vi "Periodic Tasks.vi"(8 "error in":errorcluster) -> ()   [LabVIEW 2015]
doc: "This VI runs in parallel to other tasks. It can contain as many user-defined periodic loops as you need. These can carry out PID or other sorts of timed response."
uses:
  <vilib>/Rock Robotics/WPI/Utilities/WPI_GetSetVariantRefNum.vi
  <vilib>/Rock Robotics/SystemInterfaces/Utilities/FPGA_UtilitiesRead LocalTime.vi
  <vilib>/Rock Robotics/Network Tables/NT Write Number.vi
  <vilib>/Rock Robotics/Network Tables/NT Write Numeric Array.vi
panel:
  out "All PDP Currents":dbl[](array[numeric])
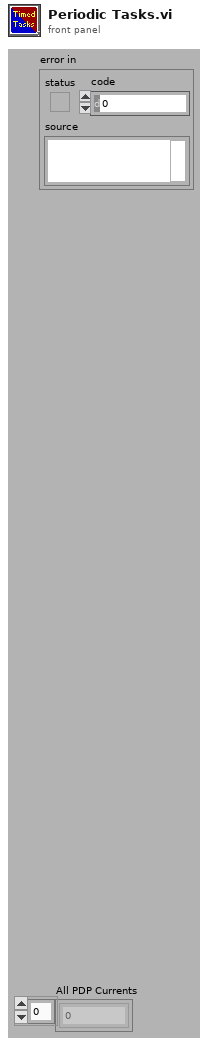
[diagram p1: front panel]
types:
  T1 = typedef "WPI_EncoderDevRef.ctl" = cluster{"DevStatus":errorcluster, "EncoderIndex":T2, "CounterIndex":T3, "DistancePerCount":dbl, "Decoding Type":T4}
  T2 = typedef "FPGA_EncoderIdx.ctl" = enum8{"Enc 0", "Enc 1", "Enc 2", "Enc 3", "Enc 4", "Enc 5", "Enc 6", "Enc 7", "Invalid"}
  T3 = typedef "FPGA_CounterCtrSystemIndex.ctl" = enum8{"Ctr 0", "Ctr 1", "Ctr 2", "Ctr 3", "Ctr 4", "Ctr 5", "Ctr 6", "Ctr 7", "Invalid"}
  T4 = typedef "WPI_EncoderType.ctl" = enum16{"1x", "2x", "4x"}
  T5 = typedef "WPI_JoystickDevRef.ctl" = cluster{"Device":T6}
  T6 = typedef "WPI_JoystickDeviceEnum.ctl" = enum16{"USB 0", "USB 1", "USB 2", "USB 3", "USB 4", "USB 5"}
  T7 = typedef "WPI_GyroDevRef.ctl" = cluster{"DevStatus":errorcluster, "Analog Channel":T8, "Offset":dbl, "Gain (VoltsPerDegree/Second)":dbl, "Gyro Type":enum16{"Analog", "XRS450"}, "Handle":i32, "SPI Bus":T9, "Device Found":bool, "Sample Rate":dbl, "Calibrate On Open":bool}
  T8 = typedef "FPGA_AIChannel.ctl" = enum8{"AI 0", "AI 1", "AI 2", "AI 3", "AI MXP 0", "AI MXP 1", "AI MXP 2", "AI MXP 3", "Invalid"}
  T9 = typedef "spi_bus.ctl" = enum16{"SPI On-Board, CS0", "SPI On-Board, CS1", "SPI On-Board, CS2", "SPI On-Board, CS3", "SPI MXP", "Invalid"}
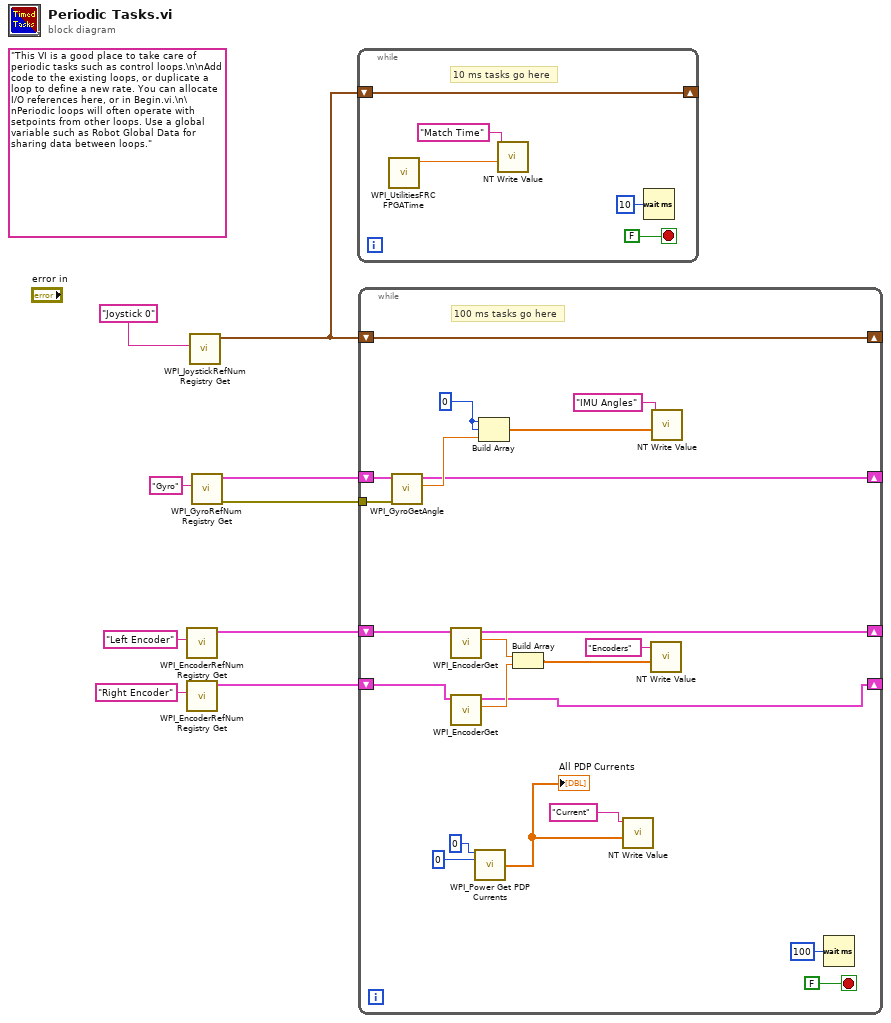
[diagram p0: block diagram]
diagram:
  (unwired) "This VI is a good place to take care of periodic tasks such as control loops.\n\nAdd code to the existing loops, or duplicate a loop to define a new rate. You can allocate I/O references here, or in Begin.vi.\n\nPeriodic loops will often operate with setpoints from other loops. Use a global variable such as Robot Global Data for sharing data between loops."
  n1 = call <vilib>:"WPI_EncoderRefNum Registry Get.vi"("refnum name"="Left Encoder") -> ("EncoderDevRef"=w5:T1)  [unwired: 9 in, 1 out]
  n2 = call <vilib>:"WPI_EncoderRefNum Registry Get.vi"("refnum name"="Right Encoder") -> ("EncoderDevRef"=w4:T1)  [unwired: 9 in, 1 out]
  n3 = call <vilib>:"WPI_JoystickRefNum Registry Get.vi"("refnum name"="Joystick 0") -> ("JoystickDevRef"=w8:T5)  [unwired: 1 in, 9 out]
  n4 = call <vilib>:"WPI_GyroRefNum Registry Get.vi"("refnum name"="Gyro") -> ("error out"=w3:errorcluster, "GyroDevRef"=w2:T7)  [unwired: 9 in]
  n5 = while {
    shift-right: [w12] -> _
    shift-left: w8 -> [w12]
    stop <- FALSE stop-if-true
    # "10 ms tasks go here"
    n6 = call <vilib>:"WPI_UtilitiesFRC FPGATime.vi"() -> ("FPGA Time"=w10:dbl)  [unwired: 10 in, 1 out]
    n7 = call-poly <vilib>:"NT Write Value.vi"("Numeric"=w10, "Name"="Match Time") -> ()  [unwired: 9 in, 1 out]
    n8 = Wait (ms)(milliseconds to wait=u32 10) -> ()  [unwired: 1 out]
  }
  n9 = while {
    shift-right: [w34] -> _
    shift-left: w8 -> [w34]
    shift-right: [w26] -> _
    shift-left: w5 -> [w28]
    shift-right: [w25] -> _
    shift-left: w4 -> [w27]
    tunnel: w3 -> [w19]
    shift-right: [w16] -> _
    shift-left: w2 -> [w15]
    stop <- FALSE stop-if-true
    w18 = 0
    # "100 ms tasks go here"
    n10 = call <vilib>:"WPI_GyroGetAngle.vi"("error in"=w19, "GyroDevRef"=w15) -> ("Angle"=w20:dbl, "GyroDevRef"=w16:T7)  [unwired: 5 in, 3 out]
    n11 = call <vilib>:"WPI_EncoderGet.vi"("EncoderDevRef"=w28) -> ("Distance"=w31:dbl, "EncoderDevRef"=w26:T1)  [unwired: 5 in, 4 out]
    n12 = call <vilib>:"WPI_EncoderGet.vi"("EncoderDevRef"=w27) -> ("Distance"=w30:dbl, "EncoderDevRef"=w25:T1)  [unwired: 5 in, 4 out]
    n13 = call <vilib>:"WPI_Power Get PDP Currents.vi"("Power Distribution Panel (0)"=u8 0, "PDP Channel"=0) -> ("all currents (A)"=w22:dbl[])  [unwired: 11 in, 2 out]
    "All PDP Currents" <- w22
    n14 = Build Array(w18, w18, w20) -> (w17:dbl[])
    n15 = Build Array(w31, w30) -> (w29:dbl[])
    n16 = call-poly <vilib>:"NT Write Value.vi"("Numeric Array"=w22, "Name"="Current") -> ()  [unwired: 9 in, 1 out]
    n17 = call-poly <vilib>:"NT Write Value.vi"("Numeric Array"=w29, "Name"="Encoders") -> ()  [unwired: 9 in, 1 out]
    n18 = call-poly <vilib>:"NT Write Value.vi"("Numeric Array"=w17, "Name"="IMU Angles") -> ()  [unwired: 9 in, 1 out]
    n19 = Wait (ms)(milliseconds to wait=u32 100) -> ()  [unwired: 1 out]
  }
